vi "IntGain.vi"(7 "Initialize?":bool, 8 "Lower Limit":fxp<+/-,25,5>[](array[numeric])=[0.0, 0.0, 0.0, 0.0], 9 "Upper Limit":fxp<+/-,25,5>[](array[numeric])=[0.0, 0.0, 0.0, 0.0], 10 "Ki*Ts":fxp<+,17,0>[](array[numeric])=[0.0, 0.0, 0.0, 0.0], 11 "Ctrl Effort In":fxp<+/-,25,5>[](array[numeric])=[0.0, 0.0, 0.0, 0.0]) -> (3 "Ctrl Effort Out":fxp<+/-,25,5>[](array[numeric]))   [LabVIEW 2020, in "Controller.lvlib"]
doc: "Implement Integral Gain, with anti-windup\nu(k) = u(k-1) + Ki*Ts*e(k)"
uses:
  Controller.lvlib
  <vilib>/Platform/TimedLoop/XDataNode/timing_clust.ctl
  <vilib>/Platform/TimedLoop/XDataNode/nitl_modes.ctl
  <vilib>/Platform/TimedLoop/XDataNode/wakeup.ctl
  <vilib>/rvi/Emulation/niFpgaSctlEmulationGetInTimedLoop.vi
  <vilib>/rvi/Emulation/niFpgaEmulationReportErrorSimple.vi
  <vilib>/rvi/Emulation/niFpgaGetClockAttributes.vi
  <vilib>/rvi/Emulation/niFpgaCriticalErrorInLSC.vi
  <vilib>/Platform/TimedLoop/XDataNode/XDataNode.xnode
  <vilib>/rvi/FXPMathLib/FxpMul/XNode/nifxpmath_Multiplier.xnode
  <vilib>/rvi/FXPMathLib/FxpAdd/XNode/nifxpmath_Add.xnode
  <vilib>/Platform/TimedLoop/XDataNode/XDNodeRunTimeDep.lvlib
  <vilib>/rvi/FXPMathLib/sim/FxpSim.dll
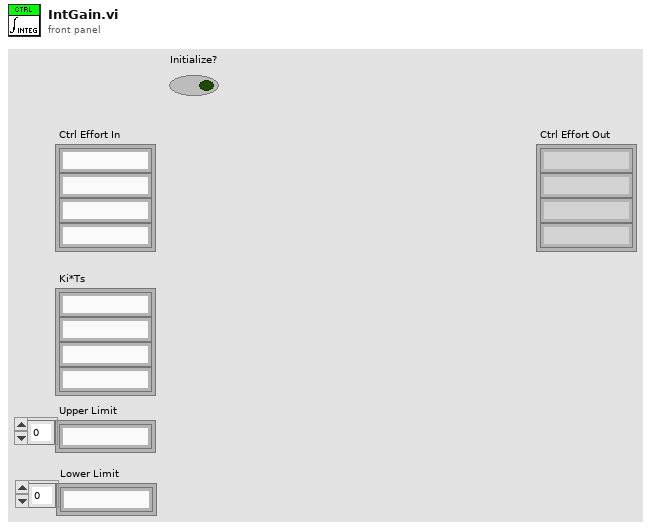
[diagram p1: front panel]
types:
  T1 = typedef "XDNodeRunTimeDep.lvlib/timing_clust.ctl" = cluster{"Expected End [f-1]":u64, "Actual End [f-1]":u64, "Finished Late? [f-1]":bool, "Expected End [i-1]":u64, "Actual End [i-1]":u64, "Finished Late? [i-1]":bool, "Expected Start [i]":u64, "Actual Start [i]":u64, "Expected Start [f]":u64, "Actual Start [f]":u64, "Source Name":string, "Structure Name":string, "Period":i64, "Deadline":i64, "Offset":i64, "Start":i64, "Priority":i32, "Timeout":i32, "Mode":T2, "Wakeup Reason":T3, "Error":errorcluster, "Source Type":string, "Secondary Source Type":string, "Global End Time":u64, "Global Start Time":u64, "Frame Duration":u64, "Iteration Duration":u64, "Assigned CPU":i32, "I/O Scan Engine Mode":u32}
  T2 = typedef "XDNodeRunTimeDep.lvlib/nitl_modes.ctl" = enum32{"No Change", "Process missed periods, maintain original phase", "Discard missed periods, maintain original phase", "Process missed periods, ignore original phase", "Discard missed periods, ignore original phase"}
  T3 = typedef "XDNodeRunTimeDep.lvlib/wakeup.ctl" = enum32{"Normal", "Aborted", "Asynchronous wakeup", "Timing source error", "Timed loop error", "Timeout"}
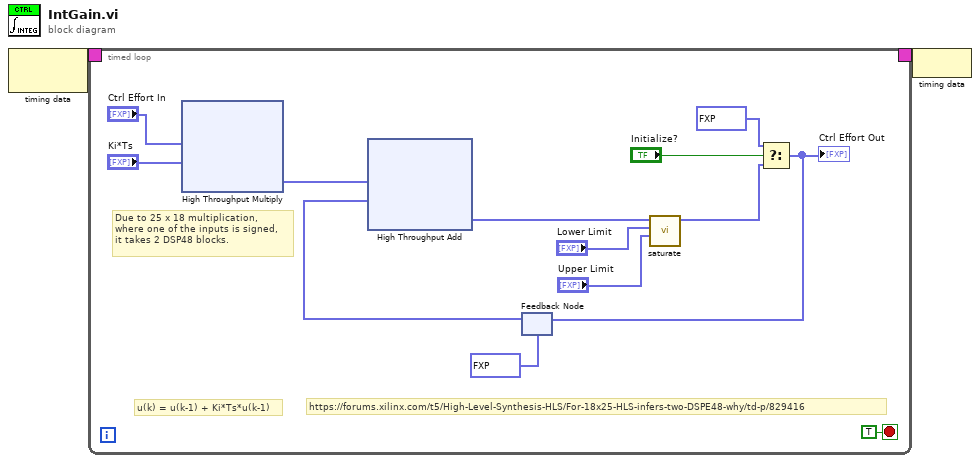
[diagram p0: block diagram]
diagram:
  n1 = node-c288() -> (w2:T1)  [unwired: 1 in]
  n2 = timed-loop {
    timing: w2 -> [_]
    timing-out: [_] -> w1
    stop <- TRUE stop-if-true
    # "https://forums.xilinx.com/t5/High-Level-Synthesis-HLS/For-18x25-HLS-infers-two-DSPE48-why/td-p/829416"
    # "Due to 25 x 18 multiplication,\nwhere one of the inputs is signed,\nit takes 2 DSP48 blocks."
    # "u(k) = u(k-1) + Ki*Ts*u(k-1)"
    n3 = xnode ("High Throughput Multiply")("x"="Ctrl Effort In", "y"="Ki*Ts") -> ("x*y"=w10:fxp<+/-,45,5>[])
    n4 = feedback #1(fxp<+/-,25,5>[] [0.0, 0.0, 0.0, 0.0] ("t")) -> (w7:fxp<+/-,25,5>[])
    n5 = xnode ("High Throughput Add")("x"=w10, "y"=w7) -> ("x+y"=w6:fxp<+/-,25,5>[])
    n6 = call "saturate.vi"("Upper Limit"="Upper Limit", "Lower Limit"="Lower Limit", "Array In"=w6) -> ("Array Out"=w3:fxp<+/-,25,5>[])  [unwired: 8 in]
    n7 = Select(t=fxp<+/-,25,5>[] [0.0, 0.0, 0.0, 0.0], s="Initialize?", f=w3) -> (s? t:f=w8:fxp<+/-,25,5>[])
    "Ctrl Effort Out" <- w8
    n8 = feedback-in #1(w8) -> ()
  }
  n9 = node-c288(w1) -> ()
